vi "Take Reading.vi"(0 "Data In":string[][](array[string]), 1 "RelHumidity":string, 2 "RoomTemp":string, 5 "Master Reading":string, 7 "Write Array":bool[](array[boolean]), 9 "Data Readings":dbl[](array[numeric]), 11 "MasterCol":i32) -> (4 "Data Out":string[][](array[string]))   [LabVIEW 2013]
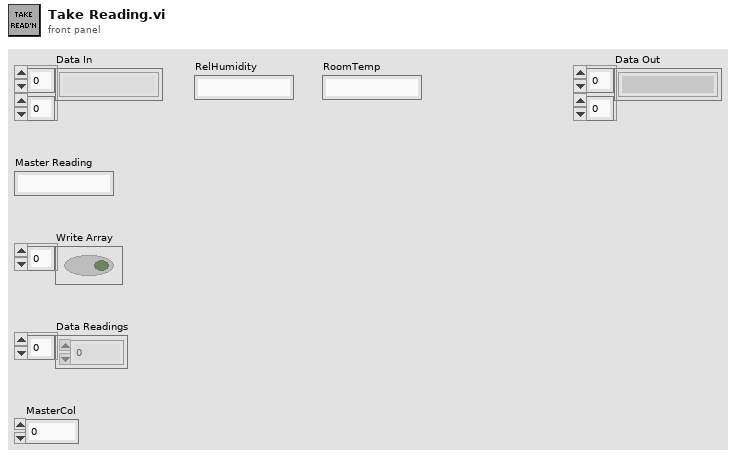
[diagram p1: front panel]
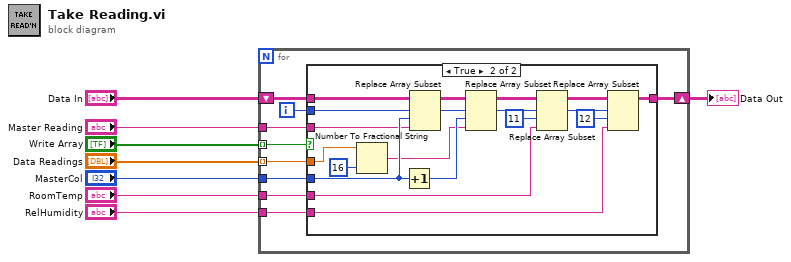
[diagram p0: block diagram]
diagram:
  n1 = for {
    tunnel: "Write Array" -> [w17] mode=indexing
    tunnel: "Data Readings" -> [w15] mode=indexing
    tunnel: "MasterCol" -> [w14]
    tunnel: "Master Reading" -> [w16]
    shift-right: [w12] -> w7
    shift-left: "Data In" -> [w13]
    tunnel: "RoomTemp" -> [w10]
    tunnel: "RelHumidity" -> [w9]
    i -> [w11]
    n2 = case shown="True" w17 {
      tunnel: w16 -> [_ w30]
      tunnel: w15 -> [_ w29]
      tunnel: w14 -> [_ w32]
      tunnel: w13 -> [w18 w34]
      tunnel: [w18 w24] -> w12
      tunnel: w11 -> [_ w23]
      tunnel: w10 -> [_ w20]
      tunnel: w9 -> [_ w19]
      frame False {
        # "Channel not selected\ndo nothing"
      }
      frame True {
        n3 = Number To Fractional String(number=w29, precision (6)=i16 16) -> (F-format string=w28:string)  [unwired: 2 in]
        n4 = Increment(x=w32) -> (x+1=w31:i32)
        n5 = Replace Array Subset(array=w34, new element=w30, index (row)=w23, index (col)=w32) -> (w33:string[][])
        n6 = Replace Array Subset(array=w33, new element=w28, index (row)=w23, index (col)=w31) -> (w26:string[][])
        n7 = Replace Array Subset(array=w26, new element=w20, index (row)=w23, index (col)=11 ("disabled index (col)")) -> (w25:string[][])
        n8 = Replace Array Subset(array=w25, new element=w19, index (row)=w23, index (col)=12 ("disabled index (col)")) -> (w24:string[][])
      }
    }
  }
  "Data Out" <- w7
